vi "Create Facade (byClass).vi"(5 "SMOFacade in":refnum<class "SMOFacade.lvclass">, 6 "Filters":string[](array[string]), 8 "error in (no error)":errorcluster, 11 "SMO":refnum<class "SMO.lvclass">) -> (0 "error out":errorcluster, 3 "SMOFacade out":refnum<class "SMOFacade.lvclass">)   [LabVIEW 2021, in "smo.lvlib" / "SMOFacade.lvclass"]
uses:
  SMOFacade.lvclass
  SMOFacade.lvclass/SMOFacade.ctl
  Registry/Registry-SMO.lvclass
  PublicEvents/PublicEvents.lvclass
  SMO/SMO.lvclass
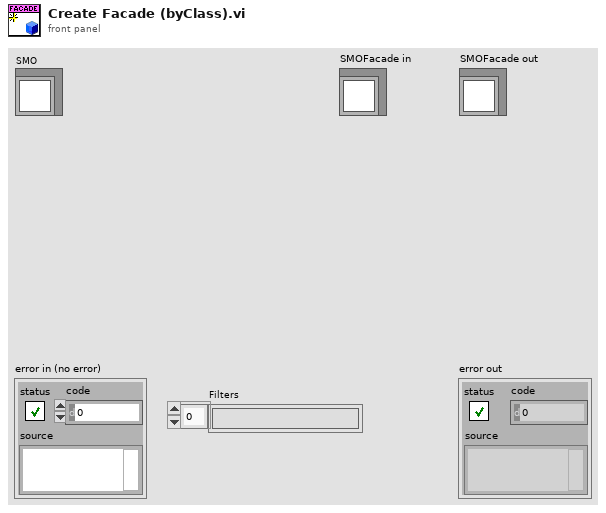
[diagram p1: front panel]
types:
  T1 = typedef "smo.lvlib/Registry-SMO.lvclass/SMO_API--Cluster.ctl" = cluster{"Method Name":string, "Full Method Name":string, "SMO Input":refnum<class "Terminal.lvclass">, "SMO Output":refnum<class "Terminal.lvclass">, "Inputs":refnum<class "Terminal.lvclass">[], "Outputs":refnum<class "Terminal.lvclass">[], "Error Output":refnum<class "Terminal.lvclass">, "vi reference":refnum<vi>}
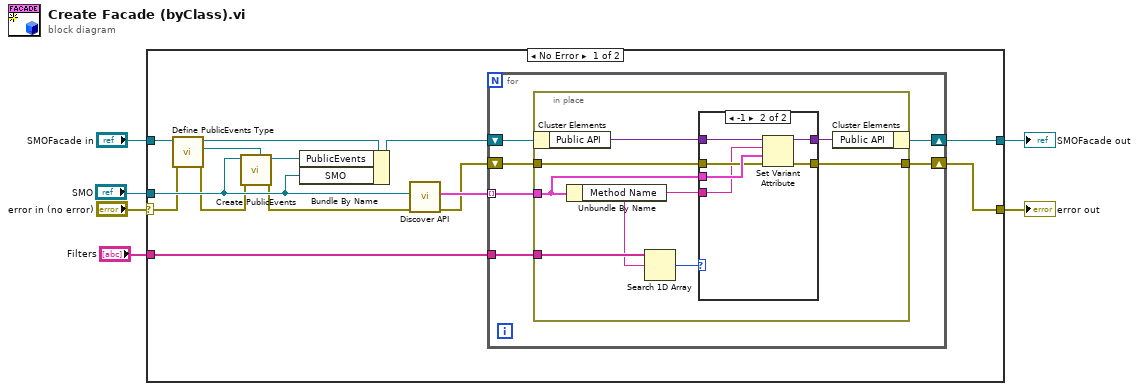
[diagram p0: block diagram]
diagram:
  n1 = case shown="No Error" "error in (no error)" {
    selector: "error in (no error)" -> [w8 w44]
    tunnel: [w16 w44] -> w5
    tunnel: [w19 w43] -> w3
    tunnel: "SMOFacade in" -> [w11 w43]
    tunnel: "SMO" -> [w14 _]
    tunnel: "Filters" -> [w15 _]
    frame No Error {
      n2 = call-dynamic "Define PublicEvents Type.vi"("error in (no error)"=w8, "SMOFacade in"=w11) -> ("error out"=w7:errorcluster, "PublicEvents type"=w9:refnum<class "PublicEvents.lvclass">, "SMOFacade out"=w10:refnum<class "SMOFacade.lvclass">)  [unwired: 7 in]
      n3 = call "Create PublicEvents.vi"("PublicEvents in"=w9, "error in (no error)"=w7, "SMO"=w14) -> ("error out"=w12:errorcluster, "PublicEvents"=w13:refnum<class "PublicEvents.lvclass">)  [unwired: 7 in]
      n4 = Bundle By Name(cluster=w10, "PublicEvents"=w13, "SMO"=w14) -> (w20:refnum<class "SMOFacade.lvclass">)
      n5 = call "Discover API.vi"("error in (no error)"=w12, "SMO"=w14) -> ("error out"=w17:errorcluster, "PublicAPI"=w18:T1[])  [unwired: 8 in]
      n6 = for {
        shift-right: [w25] -> w19
        shift-left: w20 -> [w26]
        tunnel: w18 -> [w24] mode=indexing
        shift-right: [w22] -> w16
        shift-left: w17 -> [w23]
        tunnel: w15 -> [w21]
        n7 = in-place {
          in-place-border: w24 -> [w33]
          in-place-border: w23 -> [w31]
          in-place-border: [w30] -> w22
          in-place-border: w21 -> [w29]
          n8 = in-place-cluster #1(w26) -> ("Public API"=w34:variant)
          n9 = Unbundle By Name(w33) -> ("Method Name"=w28:string)
          n10 = Search 1D Array(1D array=w29, element=w28) -> (index of element=w27:i32)  [unwired: 1 in]
          n11 = case shown="-1" w27 {
            tunnel: w34 -> [w36 w42]
            tunnel: w33 -> [_ w41]
            tunnel: [w36 w40] -> w32
            tunnel: w31 -> [w35 w39]
            tunnel: [w35 w38] -> w30
            tunnel: w28 -> [_ w37]
            frame Default {
            }
            frame -1 {
              n12 = Set Variant Attribute(Variant=w42, name=w37, value=w41, error in=w39) -> (Variant out=w40:variant, error out=w38:errorcluster)  [unwired: 1 out]
            }
          }
          n13 = in-place-cluster #1("Public API"=w32) -> (w25:refnum<class "SMOFacade.lvclass">)
        }
      }
    }
    frame Error {
    }
  }
  "error out" <- w5
  "SMOFacade out" <- w3
